vi "Default Database.vi"(8 "error in (no error)":errorcluster, 11 "Enum":enum16{"", "Default DB", "Actual DB"}(ring)=enum."Actual DB") -> (0 "error out":errorcluster)   [LabVIEW 2013, in "ConfigDBLib.lvlib"]
uses:
  ConfigDBLib.lvlib
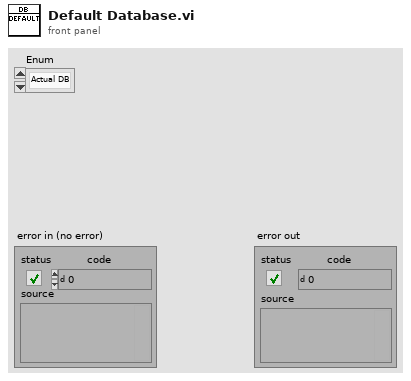
[diagram p1: front panel]
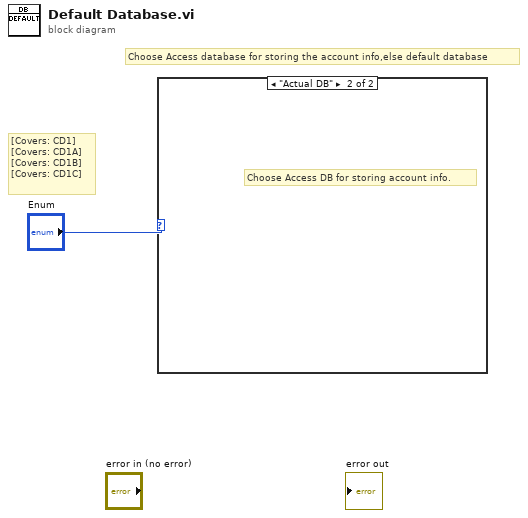
[diagram p0: block diagram]
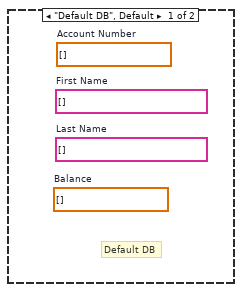
[diagram p2: hidden frame]
diagram:
  # "[Covers: CD1] \n[Covers: CD1A] \n[Covers: CD1B] \n[Covers: CD1C]"
  # "Choose Access database for storing the account info,else default database"
  n1 = case shown="\"Actual DB\"" "Enum" {
    frame "Default DB", Default {
      (unwired) dbl[] []  # Balance
      (unwired) string[] []  # Last Name
      (unwired) string[] []  # First Name
      (unwired) dbl[] []  # Account Number
      # "Default DB"
    }
    frame "Actual DB" {
      # "Choose Access DB for storing account info."
    }
  }
